vi "Query Set Temperature 9620.vi"(8 "error in (no error)":errorcluster, 11 "VISA resource name":refnum<visa-resource-name>="COM3") -> (0 "error out":errorcluster, 2 "Set temperature":dbl, 3 "VISA resource name out":refnum<visa-resource-name>)   [LabVIEW 2023]
panel:
  out "Command string":string="S"
  out "read buffer":string
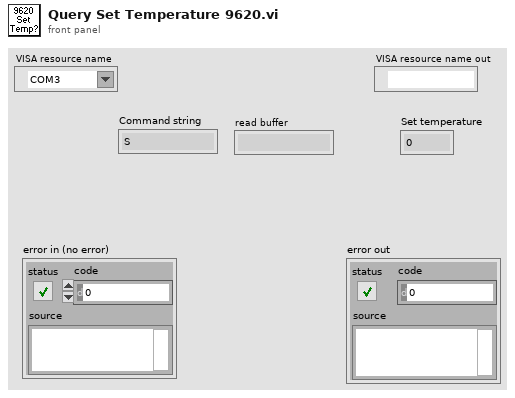
[diagram p1: front panel]
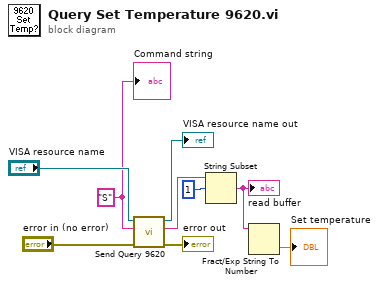
[diagram p0: block diagram]
diagram:
  w3 = "S"
  n1 = call "Send Query 9620.vi"("error in (no error)"="error in (no error)", "Query"=w3, "VISA resource name"="VISA resource name") -> ("error out"=→"error out":errorcluster, "read buffer"=w8:string, "VISA resource name out"=→"VISA resource name out":refnum<visa-resource-name>)  [unwired: 6 in]
  n2 = String Subset(string=w8, offset (0)=1) -> (substring=w2:string)  [unwired: 1 in]
  "read buffer" <- w2
  n3 = Fract/Exp String To Number(string=w2) -> (number=→"Set temperature":dbl)  [unwired: 3 in, 1 out]
  "Command string" <- w3
